vi "receiveData.vi"(8 "error in (no error)":errorcluster, 11 "Model in":refnum<class "Model.lvclass">) -> (0 "error out":errorcluster, 3 "Model out":refnum<class "Model.lvclass">)   [LabVIEW 2013, in "Model.lvclass"]
uses:
  Model.lvclass
  Typedefs/InputData.ctl
  <userlib>/Common/ILC/Typedefs/LimitSwitches.ctl
  Typedefs/ForceDemand.ctl
  Typedefs/Distance Data.ctl
  Typedefs/TemperatureData.ctl
  Model.lvclass/Model.ctl
  <userlib>/Common/ILC/ILC/ILC.lvclass/ILC.ctl
  ApplicationElements/ForceSensor/ForceSensor.lvclass/ForceSensor.ctl
  <userlib>/Common/ILC/ILC/ILC.lvclass
  ApplicationElements/DistanceGauge/DistanceGauge.lvclass
  ApplicationElements/TemperatureSensor/TemperatureSensor/TemperatureSensor.lvclass
  ApplicationElements/ForceSensor/ForceSensor.lvclass
  <userlib>/Common/ILC/Typedefs/ILCTypedefs.lvlib
  Typedefs/M2AADTTypedefs.lvlib
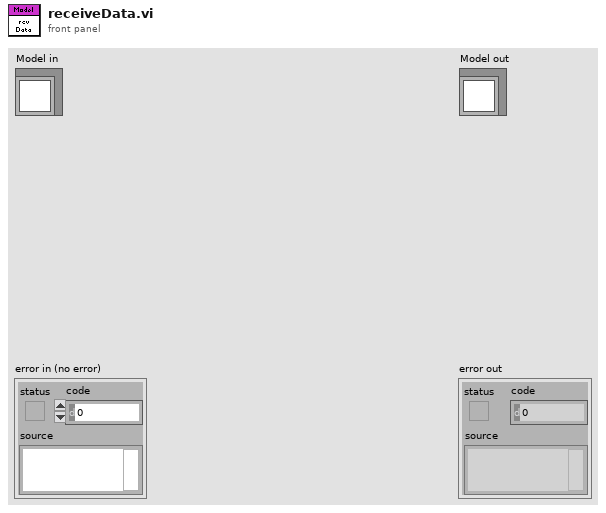
[diagram p1: front panel]
types:
  T1 = typedef "M2AADTTypedefs.lvlib/TemperatureData.ctl" = cluster{"Ambient Temperature":dbl[unit], "Motor Temperature":dbl[unit]}
  T2 = typedef "M2AADTTypedefs.lvlib/InputData.ctl" = cluster{"Limit Switches":T3, "SSI Encoder":i32, "Force Measured":T4, "Distance Data":T5, "Temperature Data":T1}
  T3 = typedef "ILCCommon.lvlib/ILCTypedefs.lvlib/LimitSwitches.ctl" = cluster{"1":bool, "2":bool}
  T4 = typedef "M2AADTTypedefs.lvlib/ForceDemand.ctl" = dbl[unit]
  T5 = typedef "M2AADTTypedefs.lvlib/Distance Data.ctl" = cluster{"Distance Measured 1":dbl[unit], "Distance Measured 2":dbl[unit]}
  T6 = typedef "ILCCommon.lvlib/ILCTypedefs.lvlib/ADCsInEngineeringUnits.ctl" = cluster{"Ch1":dbl[unit], "Ch2":dbl[unit], "Ch3":dbl[unit], "Ch4":dbl[unit], "Ch5":dbl[unit]}
  T7 = typedef "ILCCommon.lvlib/ILCTypedefs.lvlib/InputData.ctl" = cluster{"Input Channels":T8, "Limit Switches":T3, "Tachometer":u16, "SSI Encoder":i32, "ADCs":T9}
  T8 = typedef "ILCCommon.lvlib/ILCConfiguration.lvlib/InputChannels.ctl" = enum16{"Channel 0", "3 Channels", "5 Channels"}
  T9 = typedef "ILCCommon.lvlib/ILCTypedefs.lvlib/ADCs.ctl" = cluster{"Ch1":i32, "Ch2":i32, "Ch3":i32, "Ch4":i32, "Ch5":i32}
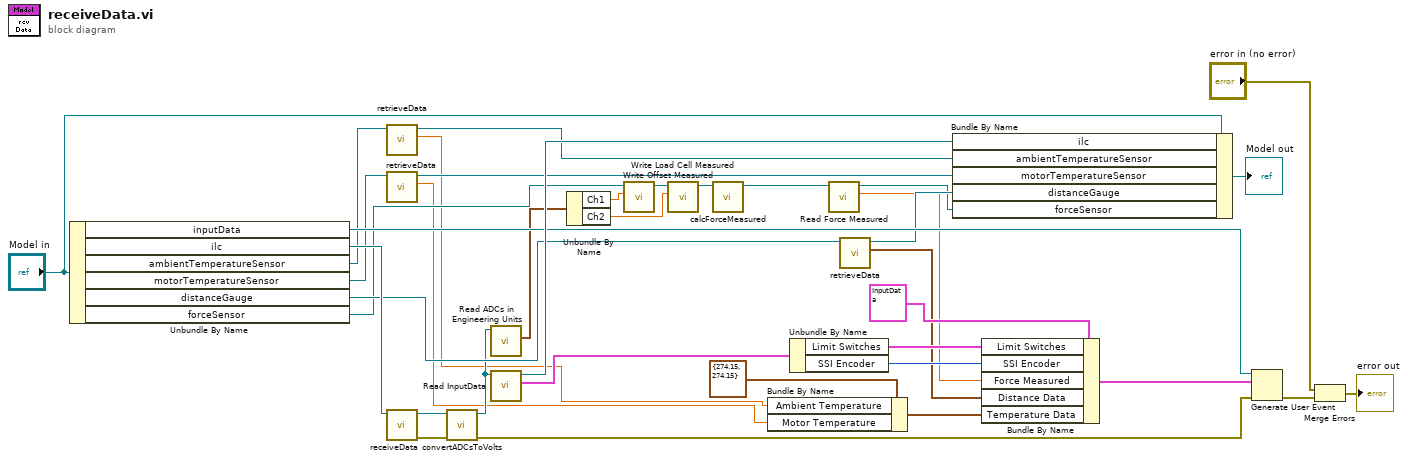
[diagram p0: block diagram]
diagram:
  n1 = Unbundle By Name("Model in") -> ("inputData"=w33:refnum<user-event>, "ilc"=w35:refnum<class "ILC.lvclass">, "ambientTemperatureSensor"=w27:refnum<class "AmbientTemperatureSensor.lvclass">, "motorTemperatureSensor"=w25:refnum<class "MotorTemperatureSensor.lvclass">, "distanceGauge"=w32:refnum<class "DistanceGauge.lvclass">, "forceSensor"=w23:refnum<class "ForceSensor.lvclass">)
  n2 = call "retrieveData.vi"("TemperatureSensor in"=w27) -> ("Temperature Measured"=w2:dbl[unit], "TemperatureSensor out"=w26:refnum<class "AmbientTemperatureSensor.lvclass">)  [unwired: 8 in, 1 out]
  n3 = call "retrieveData.vi"("TemperatureSensor in"=w25) -> ("Temperature Measured"=w1:dbl[unit], "TemperatureSensor out"=w24:refnum<class "MotorTemperatureSensor.lvclass">)  [unwired: 8 in, 1 out]
  n4 = call <userlib>:"receiveData.vi"("ILC in"=w35) -> ("error out"=w20:errorcluster, "ILC out"=w21:refnum<class "ILC.lvclass">)  [unwired: 9 in]
  n5 = call <userlib>:"convertADCsToVolts.vi"("error in (no error)"=w20, "ILC in"=w21) -> ("error out"=w19:errorcluster, "ILC out"=w18:refnum<class "ILC.lvclass">)  [unwired: 8 in]
  n6 = call <userlib>:"Read ADCs in Engineering Units.vi"("ILC in"=w18) -> ("ADCs in Engineering Units"=w17:T6)  [unwired: 9 in, 1 out]
  n7 = call <userlib>:"Read InputData.vi"("ILC in"=w18) -> ("InputData"=w9:T7, "ILC out"=w34:refnum<class "ILC.lvclass">)  [unwired: 9 in]
  n8 = Unbundle By Name(w17) -> ("Ch1"=w16:dbl[unit], "Ch2"=w15:dbl[unit])
  n9 = call "Write Offset Measured.vi"("Offset Measured"=w16, "ForceSensor in"=w23) -> ("ForceSensor out"=w22:refnum<class "ForceSensor.lvclass">)  [unwired: 9 in]
  n10 = call "Write Load Cell Measured.vi"("Load Cell Measured"=w15, "ForceSensor in"=w22) -> ("ForceSensor out"=w14:refnum<class "ForceSensor.lvclass">)  [unwired: 9 in]
  n11 = call "calcForceMeasured.vi"("ForceSensor in"=w14) -> ("ForceSensor out"=w13:refnum<class "ForceSensor.lvclass">)  [unwired: 9 in, 1 out]
  n12 = Bundle By Name(cluster=T1 {"Ambient Temperature"=274.15, "Motor Temperature"=274.15} ("Temperature Data"), "Ambient Temperature"=w2, "Motor Temperature"=w1) -> (w3:T1)
  n13 = Unbundle By Name(w9) -> ("Limit Switches"=w8:T3, "SSI Encoder"=w7:i32)
  n14 = call "Read Force Measured.vi"("ForceSensor in"=w13) -> ("Force Demand"=w6:T4, "ForceSensor out"=w12:refnum<class "ForceSensor.lvclass">)  [unwired: 9 in]
  n15 = call "retrieveData.vi"("DistanceGauge in"=w32) -> ("Distance Data"=w5:T5, "DistanceGauge out"=w31:refnum<class "DistanceGauge.lvclass">)  [unwired: 8 in, 1 out]
  n16 = Bundle By Name(cluster="Model in", "ilc"=w34, "ambientTemperatureSensor"=w26, "motorTemperatureSensor"=w24, "distanceGauge"=w31, "forceSensor"=w12) -> (→"Model out":refnum<class "Model.lvclass">)
  n17 = Bundle By Name(cluster=T2 {"Limit Switches"={"1"=FALSE, "2"=FALSE}, "SSI Encoder"=0, "Force Measured"=0.0, "Distance Data"={"Distance Measured 1"=1.0, "Distance Measured 2"=1.0}, "Temperature Data"={"Ambient Temperature"=274.15, "Motor Temperature"=274.15}} ("event data"), "Limit Switches"=w8, "SSI Encoder"=w7, "Force Measured"=w6, "Distance Data"=w5, "Temperature Data"=w3) -> (w10:T2)
  n18 = Generate User Event(user event=w33, event data cluster=w10, error in=w19) -> (error out=w29:errorcluster)  [unwired: 1 in, 1 out]
  n19 = Merge Errors("error in (no error)", w29) -> (→"error out":errorcluster)
